vi "machine_thread_states.vi"() -> (0 "error out":errorcluster, 3 "Notifier out":refnum<notifier>)   [LabVIEW 2013]
uses:
  main_machine/type_defs/data_message.ctl
  main_machine/type_defs/hts_message.ctl
  main_machine/type_defs/led_mm.ctl
  main_machine/type_defs/machine_thread_mm.ctl
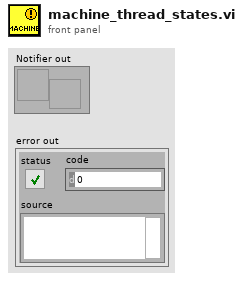
[diagram p1: front panel]
types:
  T1 = typedef "machine_thread_mm.ctl" = cluster{"DATA THREAD":T2, "HTS THREAD":T3, "LED THREAD":T4}
  T2 = typedef "data_message.ctl" = enum16{"INITIALIZE", "UPDATE DATA", "THROW AWAY DATA", "ANALYZE DATA", "SAVE DATA", "SHUTDOWN"}
  T3 = typedef "hts_message.ctl" = enum16{"INITIALIZE", "REMOVE CULTURE", "DILUTE AND INDUCE", "SAMPLE REACTOR", "CLEAR LINES", "MOVE TO NEXT", "SHUTDOWN"}
  T4 = typedef "led_mm.ctl" = enum16{"INITALIZE", "START LEDS", "STROBE", "SHUTDOWN"}
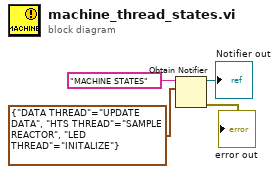
[diagram p0: block diagram]
diagram:
  n1 = Obtain Notifier(name (unnamed)="MACHINE STATES", notification data type=T1 {"DATA THREAD"=enum."UPDATE DATA", "HTS THREAD"=enum."SAMPLE REACTOR", "LED THREAD"=enum."INITALIZE"} ("output cluster")) -> (notifier out=→"Notifier out":refnum<notifier>, error out=→"error out":errorcluster)  [unwired: 2 in, 1 out]
